vi "Get-delayed-path-data.vi"(8 "error in (no error)":errorcluster, 10 "File path":path) -> (0 "error out":errorcluster, 2 "Formatted contents":string)   [LabVIEW 2013, in "HardwareCharacterization.lvlib" / "HC-SM1000.lvclass"]
uses:
  HC-SM1000.lvclass
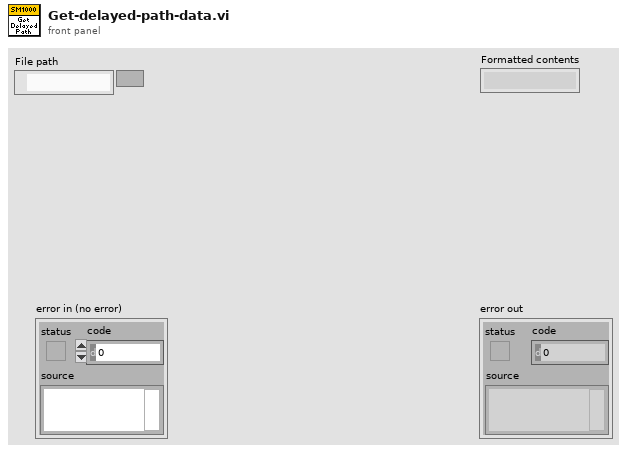
[diagram p1: front panel]
types:
  T1 = enum16{"open", "replace", "create", "open or create", "replace or create", "replace or create with confirmation"}
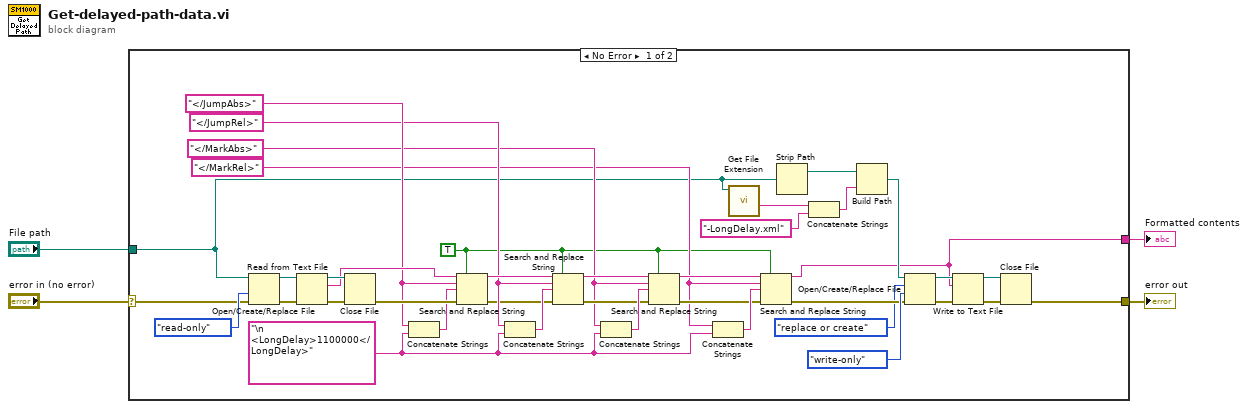
[diagram p0: block diagram]
diagram:
  n1 = case shown="No Error" "error in (no error)" {
    selector: "error in (no error)" -> [w13 w44]
    tunnel: [w12 w44] -> w3
    tunnel: "File path" -> [w7 _]
    tunnel: [w9 _] -> w1
    frame No Error {
      w10 = TRUE
      w23 = "</MarkRel>" ("search string")
      w28 = "</MarkAbs>" ("search string")
      w33 = "</JumpRel>" ("search string")
      w24 = "\n  <LongDelay>1100000</LongDelay>" ("search string")
      w36 = "</JumpAbs>" ("search string")
      n2 = Open/Create/Replace File(file path (use dialog)=w7, error in=w13, access (0:read/write)=enum16{"read/write", "read-only", "write-only"}."read-only") -> (refnum out=w43:refnum<file>, error out=w40:errorcluster)  [unwired: 3 in, 1 out]
      n3 = Read from Text File(file (use dialog)=w43, error in=w40) -> (refnum out=w42:refnum<file>, text=w38:string, error out=w41:errorcluster)  [unwired: 2 in, 1 out]
      n4 = Close File(refnum=w42, error in=w41) -> (error out=w39:errorcluster)  [unwired: 1 out]
      n5 = Concatenate Strings(w36, w24) -> (w37:string)
      n6 = Search and Replace String(replace all?=w10, input string=w38, search string=w36, replace string=w37, error in=w39) -> (result string=w34:string, error out=w32:errorcluster)  [unwired: 3 in, 2 out]
      n7 = Concatenate Strings(w33, w24) -> (w35:string)
      n8 = Search and Replace String(replace all?=w10, input string=w34, search string=w33, replace string=w35, error in=w32) -> (result string=w30:string, error out=w29:errorcluster)  [unwired: 3 in, 2 out]
      n9 = Concatenate Strings(w28, w24) -> (w31:string)
      n10 = Search and Replace String(replace all?=w10, input string=w30, search string=w28, replace string=w31, error in=w29) -> (result string=w26:string, error out=w25:errorcluster)  [unwired: 3 in, 2 out]
      n11 = Concatenate Strings(w23, w24) -> (w27:string)
      n12 = call <vilib>:"Get File Extension.vi"("file"=w7) -> ("filename without extension"=w6:string)  [unwired: 7 in, 3 out]
      n13 = Search and Replace String(replace all?=w10, input string=w26, search string=w23, replace string=w27, error in=w25) -> (result string=w9:string, error out=w11:errorcluster)  [unwired: 3 in, 2 out]
      n14 = Strip Path(path=w7) -> (stripped path=w16:path)  [unwired: 1 out]
      n15 = Concatenate Strings(w6, "-LongDelay.xml" ("string")) -> (w15:string)
      n16 = Build Path(base path=w16, name or relative path=w15) -> (appended path=w14:path)
      n17 = Open/Create/Replace File(file path (use dialog)=w14, error in=w11, operation (0:open)=T1."replace or create", access (0:read/write)=enum16{"read/write", "read-only", "write-only"}."write-only") -> (refnum out=w21:refnum<file>, error out=w18:errorcluster)  [unwired: 2 in, 1 out]
      n18 = Write to Text File(file (use dialog)=w21, text=w9, error in=w18) -> (refnum out=w20:refnum<file>, error out=w19:errorcluster)  [unwired: 1 in, 1 out]
      n19 = Close File(refnum=w20, error in=w19) -> (error out=w12:errorcluster)  [unwired: 1 out]
    }
    frame Error {
    }
  }
  "error out" <- w3
  "Formatted contents" <- w1
